vi "send add search paths.vi"(8 "error in":errorcluster, 10 "search paths":cluster{"tokenized path":T1}[](array[cluster]), 11 "message queue in":T2) -> (0 "error out":errorcluster, 3 "message queue out":T2)   [LabVIEW 2013, in "module execution process.lvlib"]
uses:
  module execution process.lvlib
  <vilib>/NI/AMC/Message Queue.ctl
  <vilib>/NI/AMC/Message.ctl
  <vilib>/NI/Tools/Keyed Array/KeyedArray.ctl
  tokenized path.ctl
  command commands to rtexe process.ctl
  <vilib>/NI/AMC/Create Single Message.vi
  <vilib>/NI/AMC/Update Message Routing Info.vi
  <vilib>/NI/AMC/Send Message.vi
  <vilib>/NI/AMC/AMC.lvlib
  <vilib>/NI/Tools/Keyed Array/Tools_KeyedArray.lvlib
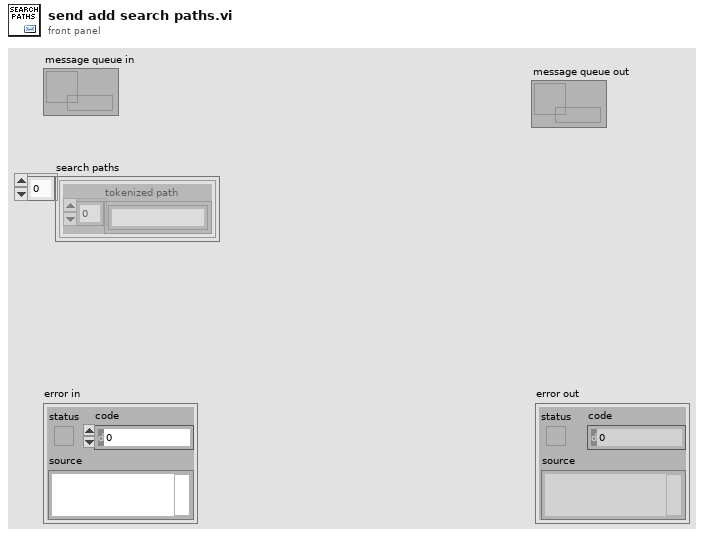
[diagram p1: front panel]
types:
  T1 = typedef "module execution process.lvlib/tokenized path.ctl" = string[]
  T2 = typedef "AMC.lvlib/Message Queue.ctl" = refnum<queue>
  T3 = typedef "module execution process.lvlib/command commands to rtexe process.ctl" = enum16{"Initialize", "Load from File", "Load from String", "Open All Engines", "Open Single Engine", "Initialize All Engines", "Initialize Single Engine", "Start All", "Start Single", "Pause All", "Pause Single", "Stop All", "Stop Single", "Close All", "Close Single", "Set Safe State All", "Set Safe State Single", "Get Status", "Exit", "Error", "Load Bitfile", "Unload Bitfile", "Add Search Paths"}
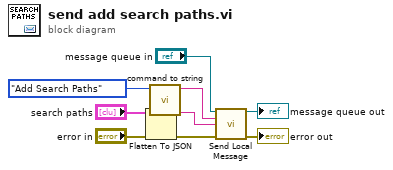
[diagram p0: block diagram]
diagram:
  n1 = Flatten To JSON(anything="search paths", error in (no error)="error in") -> (JSON string=w2:string, 11:w3:errorcluster)  [unwired: 1 in]
  n2 = call "command to string.vi"("commands"=command_commands_to_rtexe_process."Add Search Paths") -> ("command string"=w5:string)  [unwired: 10 in]
  n3 = call <vilib>:"Send Local Message.vi"("message queue in"="message queue in", "message name"=w5, "message value"=w2, "error in"=w3) -> ("message queue out"=→"message queue out":T2, "error out"=→"error out":errorcluster)  [unwired: 9 in, 1 out]
